vi "GE5565 Close (Cluster) mod.vi"(4 "error in (no error)":errorcluster, 7 "VMIC reference in":T1) -> (0 "error out":errorcluster)   [LabVIEW 2019, in "RefMem DMA Engine.lvlib"]
uses:
  RefMem DMA Engine.lvlib
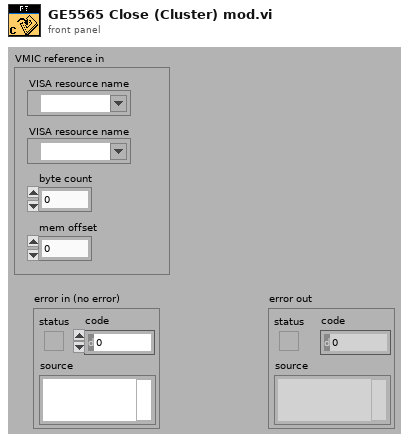
[diagram p1: front panel]
types:
  T1 = cluster{"VISA resource name":refnum<visa-resource-name>, "VISA resource name":refnum<visa-resource-name>, "byte count":u32, "mem offset":u32}
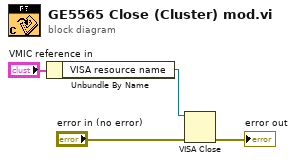
[diagram p0: block diagram]
diagram:
  n1 = Unbundle By Name("VMIC reference in") -> ("VISA resource name"=w1:refnum<visa-resource-name>)
  n2 = VISA Close(VISA resource name=w1, error in (no error)="error in (no error)") -> (error out=→"error out":errorcluster)
